vi "ENS210_ReadI2C.vi"(6 "error in (no error)":errorcluster, 8 "Byte Count":u32, 9 "Slave Address (7-bit)":u8) -> (0 "error out":errorcluster, 3 "Bytes Read":u8[](array[numeric]))   [LabVIEW 2016]
doc: "Writes data to or reads data from an Inter-Integrated Circuit (I2C) slave device through the I2C channels.\n--------------------\n\nThis Express VI is configured as follows:\n\nNode name: Pressure Sensor\nChannel: A/I2C\nMode: Read\nSpeed: Fast mode (400 kbps)"
uses:
  <vilib>/myRIO/Instrument Drivers/Onboard IO/I2C/typedefs/I2C User Configuration.ctl
  <vilib>/myRIO/Instrument Drivers/Onboard IO/I2C/typedefs/I2C Transfer Rate.ctl
  <vilib>/myRIO/Common/Instrument Driver Framework/myRIO v1.0/I2C/vis/myRIO v1.0 Read I2C.vi
  <vilib>/Utility/error.llb/Error Cluster From Error Code.vi
  <vilib>/myRIO/Common/Instrument Driver Framework/myRIO v1.0/I2C/vis/myRIO v1.0 Configure I2C.vi
  <vilib>/myRIO/Instrument Drivers/Onboard IO/I2C/I2C.lvlib
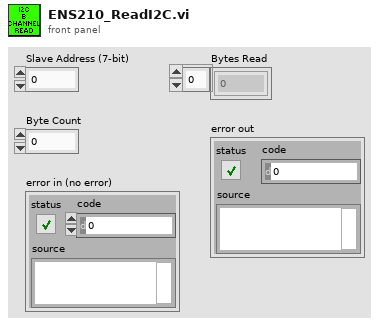
[diagram p1: front panel]
types:
  T1 = typedef "I2C.lvlib/I2C User Configuration.ctl" = cluster{"I2C Transfer Rate":T2}
  T2 = typedef "I2C.lvlib/I2C Transfer Rate.ctl" = enum16{"Standard mode (100 kbps)", "Fast mode (400 kbps)"}
  T3 = typedef "I2C.lvlib/I2C Reference.ctl" = cluster{"myRIO Reference":T4, "I2C Channels Enum":T8, "I2C Configuration":T9}
  T4 = typedef "myRIO Generic Hardware Reference.ctl" = cluster{"myRIO Model":T5, "myRIO Hardware Reference":T6}
  T5 = typedef "Hardware Version Enum.ctl" = enum16{"Unknown", "myRIO-1900", "myRIO-1950", "roboRIO", "NI ELVIS RIO CM"}
  T6 = typedef "myRIO v1.0 Reference.ctl" = cluster{"Generic FPGA Reference":T7, "Allow multiple opens":bool}
  T7 = typedef "Generic FPGA Reference.ctl" = refnum<k20>
  T8 = typedef "I2C Channels Enum.ctl" = enum16{"Not Connected", "A/I2C", "B/I2C", "I2C/I2C"}
  T9 = typedef "I2C.lvlib/I2C Configuration.ctl" = cluster{"I2C Transfer Rate":T2}
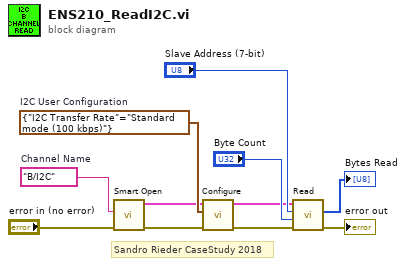
[diagram p0: block diagram]
diagram:
  w10 = T1 {"I2C Transfer Rate"=enum."Standard mode (100 kbps)"}  # I2C User Configuration
  w11 = tag "B/I2C"  # Channel Name
  # "Sandro Rieder CaseStudy 2018"
  n1 = call <vilib>:"Smart Open.vi"("error in (no error)"="error in (no error)", "Channel Name"=w11) -> ("error out"=w4:errorcluster, "I2C Ref Out"=w5:T3)  [unwired: 8 in]
  n2 = call <vilib>:"Configure.vi"("error in (no error)"=w4, "I2C User Configuration"=w10, "I2C Ref In"=w5) -> ("error out"=w2:errorcluster, "I2C Ref Out"=w3:T3)  [unwired: 7 in]
  n3 = call <vilib>:"Read.vi"("error in (no error)"=w2, "Byte Count"="Byte Count", "Slave Address (7-bit)"="Slave Address (7-bit)", "I2C Ref In"=w3) -> ("error out"=→"error out":errorcluster, "Bytes Read"=→"Bytes Read":u8[])  [unwired: 4 in, 1 out]
